vi "Read_Data.vi"(6 "Bits in Register":u8, 7 "Read Pin Task In":refnum<k21>, 8 "Clear Pin Task In":refnum<k21>, 9 "Sync Pin Task In":refnum<k21>, 10 "Data Pin Task In":refnum<k21>, 11 "Write Pin Task In":refnum<k21>) -> (0 "Clear Pin Task Out":refnum<k21>, 1 "Sync Pin Task Out":refnum<k21>, 2 "Data Pin Task Out":refnum<k21>, 3 "Write Pin Task Out":refnum<k21>, 4 "Boolean array":bool[](array[boolean]), 5 "Read Pin Task Out":refnum<k21>)   [LabVIEW 2020]
uses:
  <vilib>/DAQmx/write.llb/DAQmx Write (Digital Bool 1Line 1Point).vi
  <vilib>/DAQmx/read.llb/DAQmx Read (Digital Bool 1Line 1Point).vi
  <vilib>/DAQmx/miscellaneous.llb/DAQmx Fill In Error Info.vi
panel:
  # "___"
  # "___"
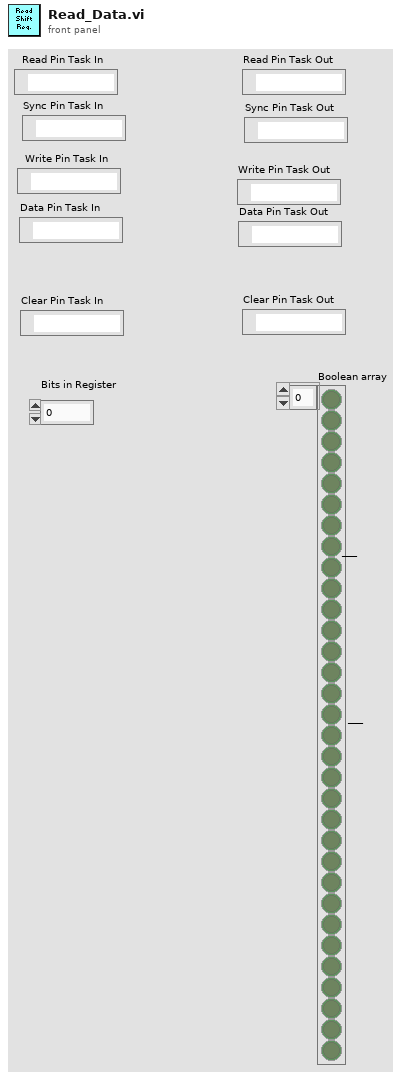
[diagram p1: front panel]
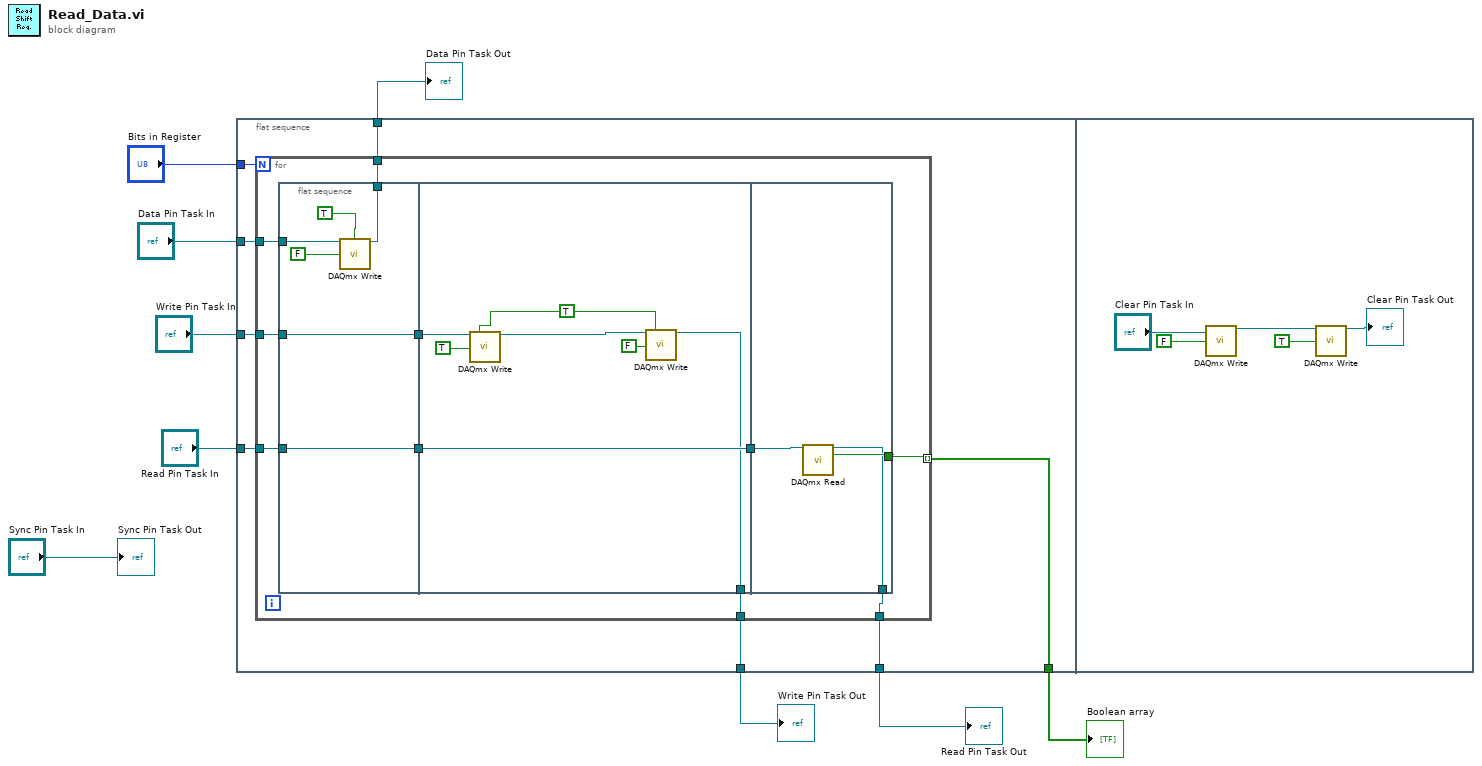
[diagram p0: block diagram]
diagram:
  n1 = flat-sequence {
    tunnel: "Data Pin Task In" -> [w17]
    tunnel: "Write Pin Task In" -> [w16]
    tunnel: "Read Pin Task In" -> [w15]
    tunnel: [w14] -> w6
    tunnel: [w13] -> w5
    tunnel: [w12] -> w4
    tunnel: "Bits in Register" -> [w11]
    tunnel: [w10] -> w2
    frame #0 {
      n2 = for {
        N: w11 -> [_]
        tunnel: w17 -> [w27]
        tunnel: w16 -> [w25]
        tunnel: w15 -> [w24]
        tunnel: [w22] -> w10 mode=indexing
        tunnel: [w21] -> w14
        tunnel: [w20] -> w13
        tunnel: [w19] -> w12
        n3 = flat-sequence {
          tunnel: w27 -> [w32]
          tunnel: [w31] -> w26
          tunnel: w25 -> [w31]
          tunnel: w24 -> [w29]
          tunnel: [w29] -> w23
          tunnel: [w28] -> w19
          tunnel: w26 -> [w36]
          tunnel: [w35] -> w18
          tunnel: w23 -> [w35]
          tunnel: [w34] -> w20
          tunnel: [w42] -> w22
          tunnel: [w41] -> w21
          tunnel: w18 -> [w43]
          frame #0 {
            n4 = call-poly <vilib>:"DAQmx Write.vi"("task/channels in"=w32, "auto start"=TRUE, "data"=FALSE) -> ("task out"=w28:refnum<k21>)  [unwired: 10 in, 2 out]
          }
          frame #1 {
            w37 = TRUE
            n5 = call-poly <vilib>:"DAQmx Write.vi"("task/channels in"=w36, "auto start"=w37, "data"=TRUE) -> ("task out"=w38:refnum<k21>)  [unwired: 10 in, 2 out]
            n6 = call-poly <vilib>:"DAQmx Write.vi"("task/channels in"=w38, "auto start"=w37, "data"=FALSE) -> ("task out"=w34:refnum<k21>)  [unwired: 10 in, 2 out]
          }
          frame #2 {
            n7 = call-poly <vilib>:"DAQmx Read.vi"("task/channels in"=w43) -> ("task out"=w41:refnum<k21>, "data"=w42:bool)  [unwired: 12 in, 1 out]
          }
        }
      }
    }
    frame #1 {
      n8 = call-poly <vilib>:"DAQmx Write.vi"("task/channels in"="Clear Pin Task In", "data"=FALSE) -> ("task out"=w46:refnum<k21>)  [unwired: 11 in, 2 out]
      n9 = call-poly <vilib>:"DAQmx Write.vi"("task/channels in"=w46, "data"=TRUE) -> ("task out"=→"Clear Pin Task Out":refnum<k21>)  [unwired: 11 in, 2 out]
    }
  }
  "Write Pin Task Out" <- w5
  "Read Pin Task Out" <- w6
  "Data Pin Task Out" <- w4
  "Boolean array" <- w2
  "Sync Pin Task Out" <- "Sync Pin Task In"
